vi "Spinning Disk Control.vi"(7 "Calling VI Ref":refnum<vi>) -> ()   [LabVIEW 2020]
uses:
  <vilib>/Utility/miscctls.llb/LVPointTypeDef.ctl
  Hardware Configuration/Hardware Configuration Controls/Device Type.ctl
  Hardware Configuration/Hardware Configuration Controls/Device Function.ctl
  SD Type Defs/SD Position Names.ctl
  Device Library/Spinning Disk/Spinning Disk Polymorphic Messenger/Get Num Positions.vi
  Device Library/Spinning Disk/Spinning Disk Polymorphic Messenger/Status.vi
  Device Library/Spinning Disk/Spinning Disk Polymorphic Messenger/Home All.vi
  Device Library/Spinning Disk/Spinning Disk Polymorphic Messenger/Refresh Pos.vi
  Device Library/Spinning Disk/Spinning Disk Polymorphic Messenger/Set Disk Position.vi
  Device Library/Spinning Disk/Spinning Disk Polymorphic Messenger/Set Dichroic Position.vi
  Device Library/Spinning Disk/Spinning Disk Polymorphic Messenger/Set Filter Position.vi
  Device Library/Spinning Disk/Spinning Disk Polymorphic Messenger/Disk Off.vi
  Device Library/Spinning Disk/Spinning Disk Polymorphic Messenger/Disk On.vi
  Device Library/Spinning Disk/Spinning Disk Polymorphic Messenger/Quit.vi
panel:
  in  "Refresh Pos":bool
  in  "Home All":bool
  in  "Quit":bool
  out "Error":bool
  in  "Disk On":bool=TRUE
  in  "Filter Wheel Position":i32(ring)
  in  "Dichroic Position":i32(ring)
  in  "Disk Position":i32(ring) items=["Disk Out", "Large Spiral", "Small Spiral"]
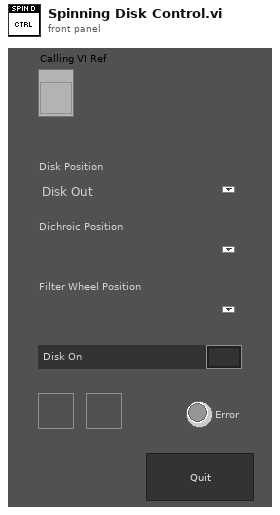
[diagram p1: front panel]
types:
  T1 = typedef "Device Function.ctl" = enum16{"Primary", "Secondary", "Overview", "Wide Field Drift Correction", "642 nm Excitation", "560 nm Excitation", "940 nm Excitation", "546 nm Excitation", "488 nm Excitation", "405 nm Excitation", "Objective Drift Correction", "4Pi Objective Lock", "Objective XY", "Objective Z", "Sample XY", "Sample Coarse Z", "Sample Z", "4Pi Lower", "4Pi Upper", "Mojo", "Adj Cavity", "Line Scanning", "Alert"}
  T2 = typedef "Device Type.ctl" = enum16{"AOTF", "Camera", "Deformable Mirror", "Laser", "Shutter", "Stage", "Waveform", "FPGA", "Email", "Filter Wheel", "Spinning Disk"}
  T3 = enum16{"Always On", "Always Off", "Off While Running"}
  T4 = typedef "LVPointTypeDef.ctl" = cluster{"Horizontal":i16, "Vertical":i16}
  T5 = typedef "SD Position Names.ctl" = cluster{"Disk Patterns":string[], "Filters":string[], "Dichroics":string[]}
  T6 = enum8{"Enabled", "Disabled", "Disabled and Grayed Out"}
  T7 = typedef "LVRectTypeDef.ctl" = cluster{"Left":i16, "Top":i16, "Right":i16, "Bottom":i16}
  T8 = typedef "LVBoundsTypeDef.ctl" = cluster{"Width":u32, "Height":u32}
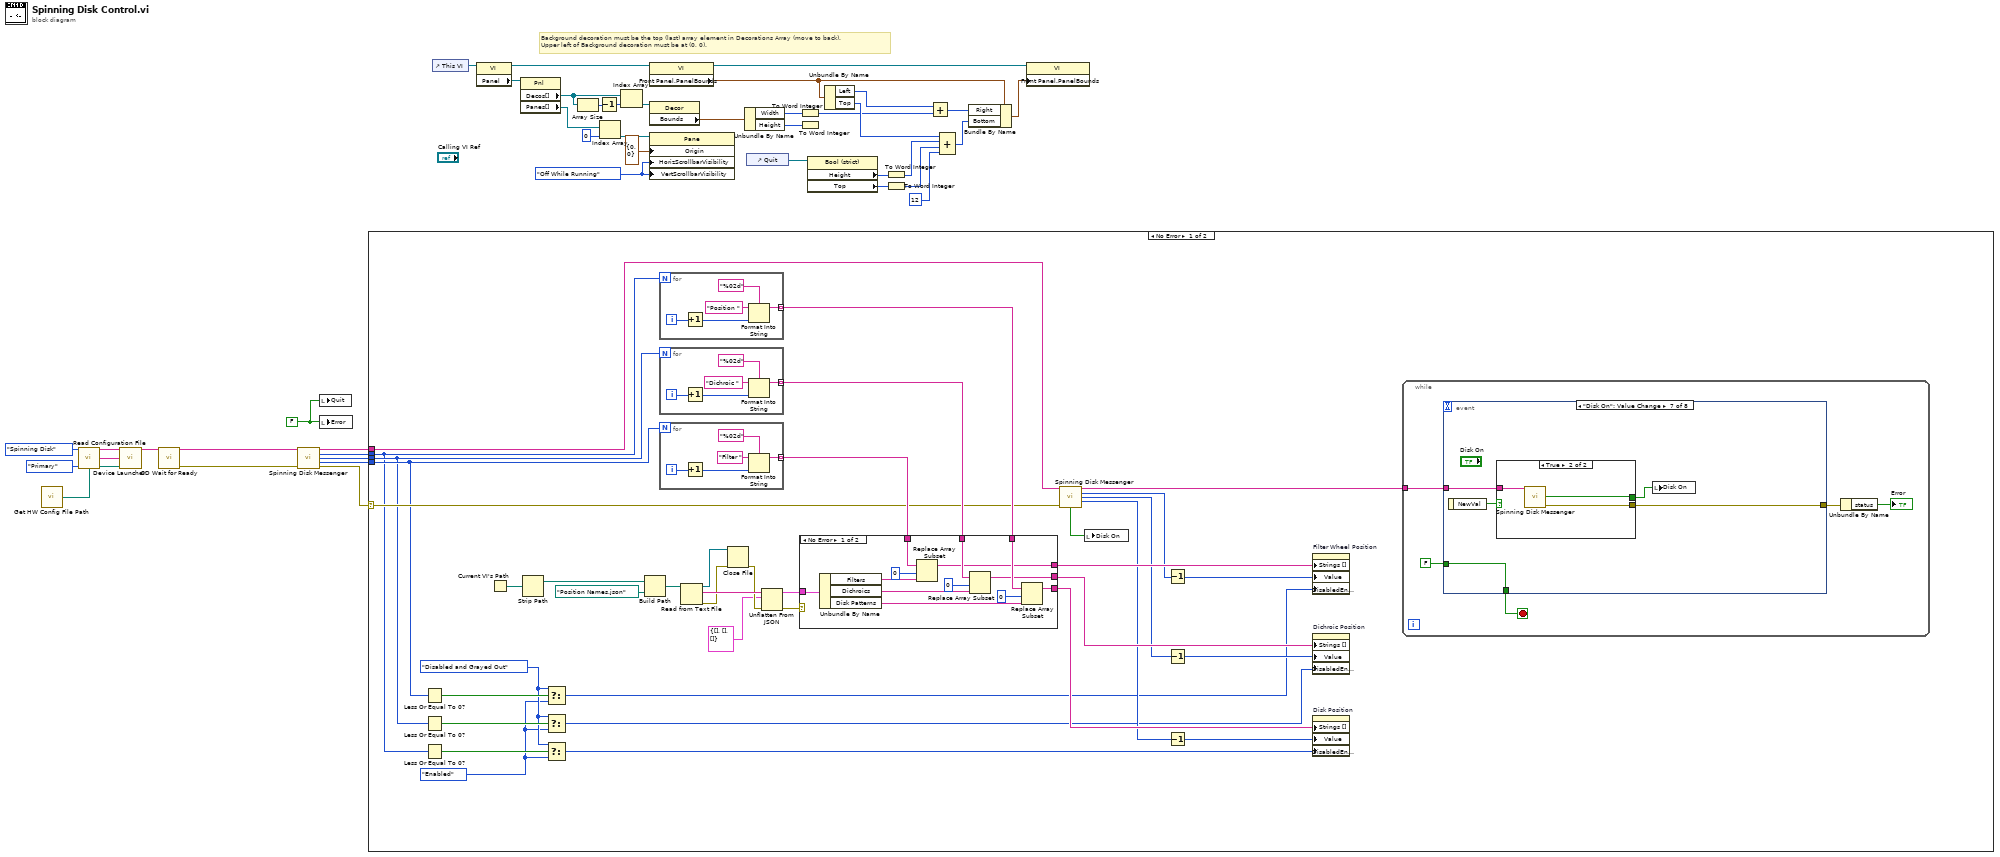
[diagram p0: block diagram]
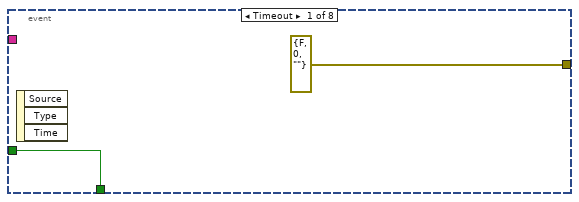
[diagram p2: hidden frame]
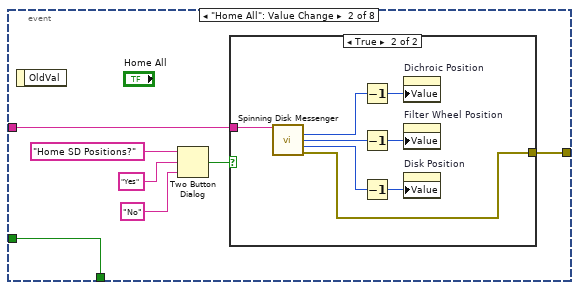
[diagram p3: hidden frame]
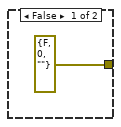
[diagram p4: hidden frame]
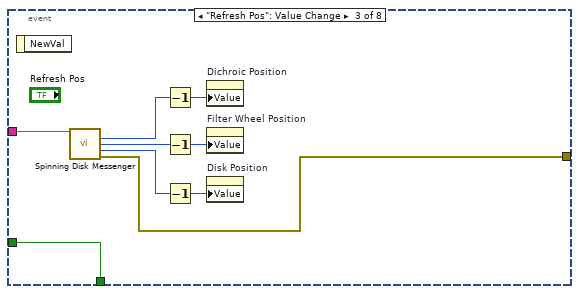
[diagram p5: hidden frame]
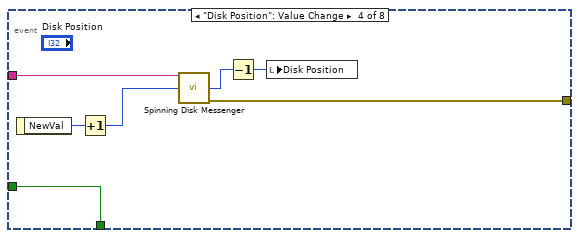
[diagram p6: hidden frame]
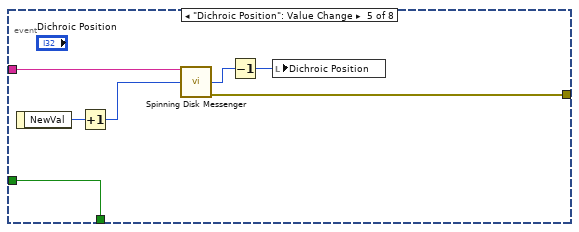
[diagram p7: hidden frame]
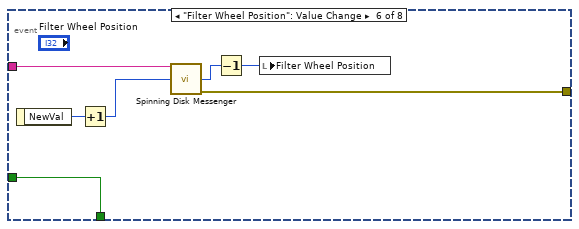
[diagram p8: hidden frame]
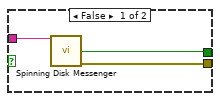
[diagram p9: hidden frame]
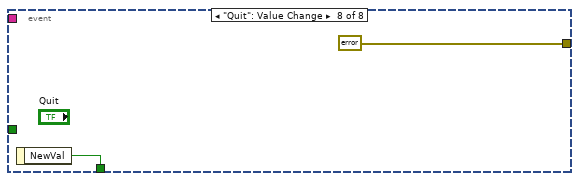
[diagram p10: hidden frame]
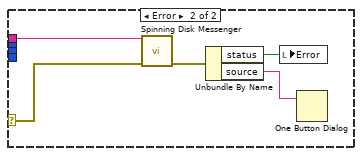
[diagram p12: hidden frame]
diagram:
  w1 = FALSE ("Error")
  w27 = T3."Off While Running" ("Vertical Scrollbar Visibility")
  # "Background decoration must be the top (last) array element in Decorations Array (move to back).\nUpper left of Background decoration must be at (0, 0)."
  n1 = call "Get HW Config File Path.vi"() -> ("File Path"=w10:path)  [unwired: 14 in, 1 out]
  n2 = call "Read Configuration File.vi"("Device Type"=Device_Type."Spinning Disk", "Device Function"=Device_Function."Primary", "Config File Path"=w10) -> ("Unique Notifier Name"=w15:string, "Device Ports/IDs/Channels"=w13:string[], "Device Engine Path"=w14:path)  [unwired: 9 in, 1 out]
  n3 = call "Device Launcher.vi"("Notifier Name"=w15, "Device Ports/IDs/Channels"=w13, "Device Engine Path"=w14) -> ("Notifier Name"=w9:string)  [unwired: 11 in, 1 out]
  n4 = call "SD Wait for Ready.vi"("Notifier Name"=w9) -> ("Notifier Name Out"=w8:string, "Error Out"=w7:errorcluster)  [unwired: 12 in, 1 out]
  n5 = call-poly "Spinning Disk Messenger.vi"("Notifier Name"=w8, "Error In"=w7) -> ("Notifier Name Dup"=w2:string, "Num Disk Pos"=w6:i32, "Num Dichroic Pos"=w5:i32, "Num Filter Pos"=w4:i32, "Error Out"=w3:errorcluster)  [unwired: 9 in]
  n6 = local write "Quit"(w1) -> ()
  n7 = local write "Error"(w1) -> ()
  n8 = case shown="No Error" w3 {
    selector: w3 -> [w64 w183]
    tunnel: w6 -> [w53 _]
    tunnel: w5 -> [w54 _]
    tunnel: w4 -> [w55 _]
    tunnel: w2 -> [w65 w184]
    frame No Error {
      w48 = T6."Enabled" ("Disabled")
      w49 = T6."Disabled and Grayed Out" ("Disabled")
      n9 = Less Or Equal To 0?(x=w55) -> (x <= 0?=w52:bool)
      n10 = Less Or Equal To 0?(x=w54) -> (x <= 0?=w50:bool)
      n11 = Less Or Equal To 0?(x=w53) -> (x <= 0?=w51:bool)
      n12 = Current VI's Path() -> (path=w82:path)
      n13 = Strip Path(path=w82) -> (stripped path=w81:path)  [unwired: 1 out]
      n14 = Select(t=w49, s=w52, f=w48) -> (s? t:f=w45:T6)
      n15 = Select(t=w49, s=w50, f=w48) -> (s? t:f=w46:T6)
      n16 = Select(t=w49, s=w51, f=w48) -> (s? t:f=w47:T6)
      n17 = Build Path(base path=w81, name or relative path=path "Position Names.json") -> (appended path=w79:path)
      n18 = for {
        N: w53 -> [_]
        tunnel: [w159] -> w71 mode=indexing
        i -> [w163]
        n19 = Increment(x=w163) -> (x+1=w160:i32)
        n20 = Format Into String(format string="%02d", initial string="Position ", w160) -> (resulting string=w159:string)  [unwired: 1 in, 1 out]
      }
      n21 = for {
        N: w54 -> [_]
        tunnel: [w154] -> w70 mode=indexing
        i -> [w158]
        n22 = Increment(x=w158) -> (x+1=w155:i32)
        n23 = Format Into String(format string="%02d", initial string="Dichroic ", w155) -> (resulting string=w154:string)  [unwired: 1 in, 1 out]
      }
      n24 = for {
        N: w55 -> [_]
        tunnel: [w149] -> w69 mode=indexing
        i -> [w153]
        n25 = Increment(x=w153) -> (x+1=w150:i32)
        n26 = Format Into String(format string="%02d", initial string="Filter ", w150) -> (resulting string=w149:string)  [unwired: 1 in, 1 out]
      }
      n27 = Read from Text File(file (use dialog)=w79) -> (refnum out=w77:refnum<file>, text=w78:string, error out=w76:errorcluster)  [unwired: 3 in, 1 out]
      n28 = Close File(refnum=w77, error in=w76) -> (error out=w75:errorcluster)  [unwired: 1 out]
      n29 = Unflatten From JSON(JSON string=w78, type and defaults=T5 {"Disk Patterns"=[], "Filters"=[], "Dichroics"=[]} ("SD Names"), error in (no error)=w75) -> (value=w72:T5, error out=w73:errorcluster)  [unwired: 4 in]
      n30 = case shown="No Error" w73 {
        tunnel: w72 -> [w176 _]
        tunnel: w71 -> [w175 w179]
        tunnel: w70 -> [w170 w178]
        tunnel: w69 -> [w167 w177]
        tunnel: [w166 w179] -> w68
        tunnel: [w165 w178] -> w66
        tunnel: [w164 w177] -> w67
        frame No Error {
          n31 = Unbundle By Name(w176) -> ("Filters"=w168:string[], "Dichroics"=w171:string[], "Disk Patterns"=w173:string[])
          n32 = Replace Array Subset(array=w167, new element=w168, index=0) -> (w164:string[])
          n33 = Replace Array Subset(array=w170, new element=w171, index=0) -> (w165:string[])
          n34 = Replace Array Subset(array=w175, new element=w173, index=0) -> (w166:string[])
        }
        frame Error {
        }
      }
      n35 = call-poly "Spinning Disk Messenger.vi"("Notifier Name"=w65, "Error In"=w64) -> ("Notifier Name Dup"=w62:string, "Filter Wheel"=w60:i32, "Dichroic"=w61:i32, "Disk Position"=w59:i32, "Disk On"=w63:bool)  [unwired: 8 in, 1 out]
      n36 = local write "Disk On"(w63) -> ()
      n37 = Decrement(x=w60) -> (x-1=w58:i32)
      n38 = Decrement(x=w61) -> (x-1=w57:i32)
      n39 = Decrement(x=w59) -> (x-1=w56:i32)
      n40 = property on="Filter Wheel Position" class="Ring (strict)"("Strings []"=w67, "Value"=w58, "DisabledEnum"=w45) -> ()  [unwired: 2 in, 2 out]
      n41 = property on="Dichroic Position" class="Ring (strict)"("Strings []"=w66, "Value"=w57, "DisabledEnum"=w46) -> ()  [unwired: 2 in, 2 out]
      n42 = property on="Disk Position" class="Ring (strict)"("Strings []"=w68, "Value"=w56, "DisabledEnum"=w47) -> ()  [unwired: 2 in, 2 out]
      n43 = while {
        tunnel: w62 -> [w85]
        stop <- w87 stop-if-true
        n44 = event shown="[6] \"Disk On\": Value Change" {
          selector: _ -> [_ _ _ _ _ _ _ _]
          dyn-events: _ -> [_ _ _ _ _ _ _ _]
          timeout: _ -> [_ _ _ _ _ _ _ _]
          tunnel: [w89 w96 w114 w121 w128 w135 w140 w148] -> w87
          tunnel: FALSE -> [w89 w96 w114 w121 w128 w135 w140 _]
          tunnel: w85 -> [_ w95 w113 w120 w127 w134 w139 _]
          tunnel: [errorcluster {"status"=FALSE, "code"=0, "source"=""} ("Error Out") w94 w106 w118 w125 w132 w137 errorcluster {"status"=FALSE, "code"=0, "source"=""} ("Error Out")] -> w84
          event Timeout {
            n45 = event-data() -> ()  [unwired: 1 in, 3 out]
          }
          event "Home All": Value Change {
            n46 = event-data() -> ()  [unwired: 1 in, 1 out]
            n47 = Two Button Dialog(message="Home SD Positions?", 1:"No" ("F button name (\"Cancel\")"), 2:"Yes" ("T button name (\"OK\")")) -> (T button?=w90:bool)
            n48 = case shown="True" w90 {
              tunnel: w95 -> [_ w105]
              tunnel: [errorcluster {"status"=FALSE, "code"=0, "source"=""} ("Error Out") w98] -> w94
              frame False {
              }
              frame True {
                n49 = call-poly "Spinning Disk Messenger.vi"("Notifier Name"=w105) -> ("Dichroic Pos"=w101:i32, "Filter Wheel Pos"=w100:i32, "Disk Pos"=w99:i32, "Error Out"=w98:errorcluster)  [unwired: 9 in, 2 out]
                n50 = Decrement(x=w101) -> (x-1=w103:i32)
                n51 = Decrement(x=w100) -> (x-1=w104:i32)
                n52 = Decrement(x=w99) -> (x-1=w102:i32)
                n53 = property on="Dichroic Position" class="Ring (strict)"("Value"=w103) -> ()  [unwired: 2 in, 2 out]
                n54 = property on="Filter Wheel Position" class="Ring (strict)"("Value"=w104) -> ()  [unwired: 2 in, 2 out]
                n55 = property on="Disk Position" class="Ring (strict)"("Value"=w102) -> ()  [unwired: 2 in, 2 out]
              }
            }
          }
          event "Refresh Pos": Value Change {
            n56 = event-data() -> ()  [unwired: 1 in, 1 out]
            n57 = call-poly "Spinning Disk Messenger.vi"("Notifier Name"=w113) -> ("Dichroic Pos"=w107:i32, "Filter Wheel Pos"=w109:i32, "Disk Pos"=w108:i32, "Error Out"=w106:errorcluster)  [unwired: 9 in, 2 out]
            n58 = Decrement(x=w107) -> (x-1=w111:i32)
            n59 = Decrement(x=w109) -> (x-1=w112:i32)
            n60 = Decrement(x=w108) -> (x-1=w110:i32)
            n61 = property on="Dichroic Position" class="Ring (strict)"("Value"=w111) -> ()  [unwired: 2 in, 2 out]
            n62 = property on="Filter Wheel Position" class="Ring (strict)"("Value"=w112) -> ()  [unwired: 2 in, 2 out]
            n63 = property on="Disk Position" class="Ring (strict)"("Value"=w110) -> ()  [unwired: 2 in, 2 out]
          }
          event "Disk Position": Value Change {
            n64 = event-data() -> ("NewVal"=w119:i32)  [unwired: 1 in]
            n65 = Increment(x=w119) -> (x+1=w115:i32)
            n66 = call-poly "Spinning Disk Messenger.vi"("Notifier Name"=w120, "Disk Position"=w115) -> ("Position"=w117:i32, "Error Out"=w118:errorcluster)  [unwired: 10 in, 2 out]
            n67 = Decrement(x=w117) -> (x-1=w116:i32)
            n68 = local write "Disk Position"(w116) -> ()
          }
          event "Dichroic Position": Value Change {
            n69 = event-data() -> ("NewVal"=w126:i32)  [unwired: 1 in]
            n70 = Increment(x=w126) -> (x+1=w122:i32)
            n71 = call-poly "Spinning Disk Messenger.vi"("Notifier Name"=w127, "Dichroic Position"=w122) -> ("Position"=w124:i32, "Error Out"=w125:errorcluster)  [unwired: 10 in, 2 out]
            n72 = Decrement(x=w124) -> (x-1=w123:i32)
            n73 = local write "Dichroic Position"(w123) -> ()
          }
          event "Filter Wheel Position": Value Change {
            n74 = event-data() -> ("NewVal"=w133:i32)  [unwired: 1 in]
            n75 = Increment(x=w133) -> (x+1=w129:i32)
            n76 = call-poly "Spinning Disk Messenger.vi"("Notifier Name"=w134, "Filter Position"=w129) -> ("Position"=w131:i32, "Error Out"=w132:errorcluster)  [unwired: 10 in, 2 out]
            n77 = Decrement(x=w131) -> (x-1=w130:i32)
            n78 = local write "Filter Wheel Position"(w130) -> ()
          }
          event "Disk On": Value Change {
            n79 = event-data() -> ("NewVal"=w138:bool)  [unwired: 1 in]
            n80 = case shown="True" w138 {
              tunnel: w139 -> [w143 w146]
              tunnel: [w142 w145] -> w137
              tunnel: [w141 w144] -> w136
              frame False {
                n81 = call-poly "Spinning Disk Messenger.vi"("Notifier Name"=w143) -> ("Disk On?"=w141:bool, "Error Out"=w142:errorcluster)  [unwired: 12 in, 1 out]
              }
              frame True {
                n82 = call-poly "Spinning Disk Messenger.vi"("Notifier Name"=w146) -> ("Disk On?"=w144:bool, "Error Out"=w145:errorcluster)  [unwired: 12 in, 1 out]
              }
            }
            n83 = local write "Disk On"(w136) -> ()
          }
          event "Quit": Value Change {
            n84 = event-data() -> ("NewVal"=w148:bool)  [unwired: 1 in]
          }
        }
        n85 = Unbundle By Name(w84) -> ("status"=→"Error":bool)
      }
    }
    frame Error {
      n86 = call-poly "Spinning Disk Messenger.vi"("Notifier Name"=w184, "Error In"=w183) -> ("Error Out"=w182:errorcluster)  [unwired: 12 in, 1 out]
      n87 = Unbundle By Name(w182) -> ("status"=w181:bool, "source"=w180:string)
      n88 = local write "Error"(w181) -> ()
      n89 = One Button Dialog(message=w180) -> ()  [unwired: 1 in, 1 out]
    }
  }
  n90 = control-ref of="This VI"() -> (w19:refnum<vi>)
  n91 = property class="VI"(reference=w19) -> (reference out=w28:refnum<vi>, "Panel"=w20:refnum<vi>)  [unwired: 1 in, 1 out]
  n92 = property class="Pnl"(reference=w20) -> ("Decos[]"=w18:refnum<vi>[], "Panes[]"=w24:refnum<vi>[])  [unwired: 1 in, 2 out]
  n93 = Array Size(array=w18) -> (size(s)=w16:i32)
  n94 = Decrement(x=w16) -> (x-1=w17:i32)
  n95 = Index Array(array=w24, index=0) -> (element=w23:refnum<vi>)
  n96 = Index Array(array=w18, index=w17) -> (element=w26:refnum<vi>)
  n97 = property class="VI"(reference=w28) -> (reference out=w30:refnum<vi>, "Front Panel.PanelBounds"=w31:T7)  [unwired: 1 in, 1 out]
  n98 = property class="Decor"(reference=w26) -> ("Bounds"=w29:T8)  [unwired: 1 in, 2 out]
  n99 = property class="Pane"(reference=w23, "Origin"=T4 {"Horizontal"=0, "Vertical"=0}, "HorizScrollbarVisibility"=w27, "VertScrollbarVisibility"=w27) -> ()  [unwired: 1 in, 2 out]
  n100 = Unbundle By Name(w29) -> ("Width"=w34:u32, "Height"=w37:u32)
  n101 = control-ref of="Quit"() -> (w21:refnum<vi>)
  n102 = To Word Integer(number=w34) -> (16bit integer=w36:i16)
  n103 = To Word Integer(number=w37) -> ()  [unwired: 1 out]
  n104 = property class="Bool (strict)"(reference=w21) -> ("Height"=w39:u32, "Top"=w40:i32)  [unwired: 1 in, 2 out]
  n105 = Unbundle By Name(w31) -> ("Left"=w33:i16, "Top"=w44:i16)
  n106 = To Word Integer(number=w39) -> (16bit integer=w42:i16)
  n107 = To Word Integer(number=w40) -> (16bit integer=w43:i16)
  n108 = Add(x=w33, y=w36) -> (x+y=w35:i16)
  n109 = Compound Arithmetic op=ADD(w44, w42, w43, i16 12 ("y")) -> (w38:i16)
  n110 = Bundle By Name(cluster=w31, "Right"=w35, "Bottom"=w38) -> (w32:T7)
  n111 = property class="VI"(reference=w30, "Front Panel.PanelBounds"=w32) -> ()  [unwired: 1 in, 2 out]
